vi "Periodic Tasks.vi"(8 "error in":errorcluster) -> ()   [LabVIEW 2016]
doc: "This VI runs in parallel to other tasks. It can contain as many user-defined periodic loops as you need. These can carry out PID or other sorts of timed response."
uses:
  <vilib>/Analysis/baseanly.llb/Mean (DBL).vi
  <vilib>/Rock Robotics/WPI/Utilities/WPI_GetSetVariantRefNum.vi
  LabView Programs/TestBot/global.vi
  <vilib>/Analysis/NI_AALBase.lvlib
panel:
  out "buffer":string
  out "error out 2":errorcluster
  out "X":i32
  out "Y":i32
  out "Width":i32
  out "Height":i32
  out "Area":dbl(graph)
  in  "Combo Box":string(combo)
  in  "Write":bool
  out "concatenated string":string
  in  "Flush":bool
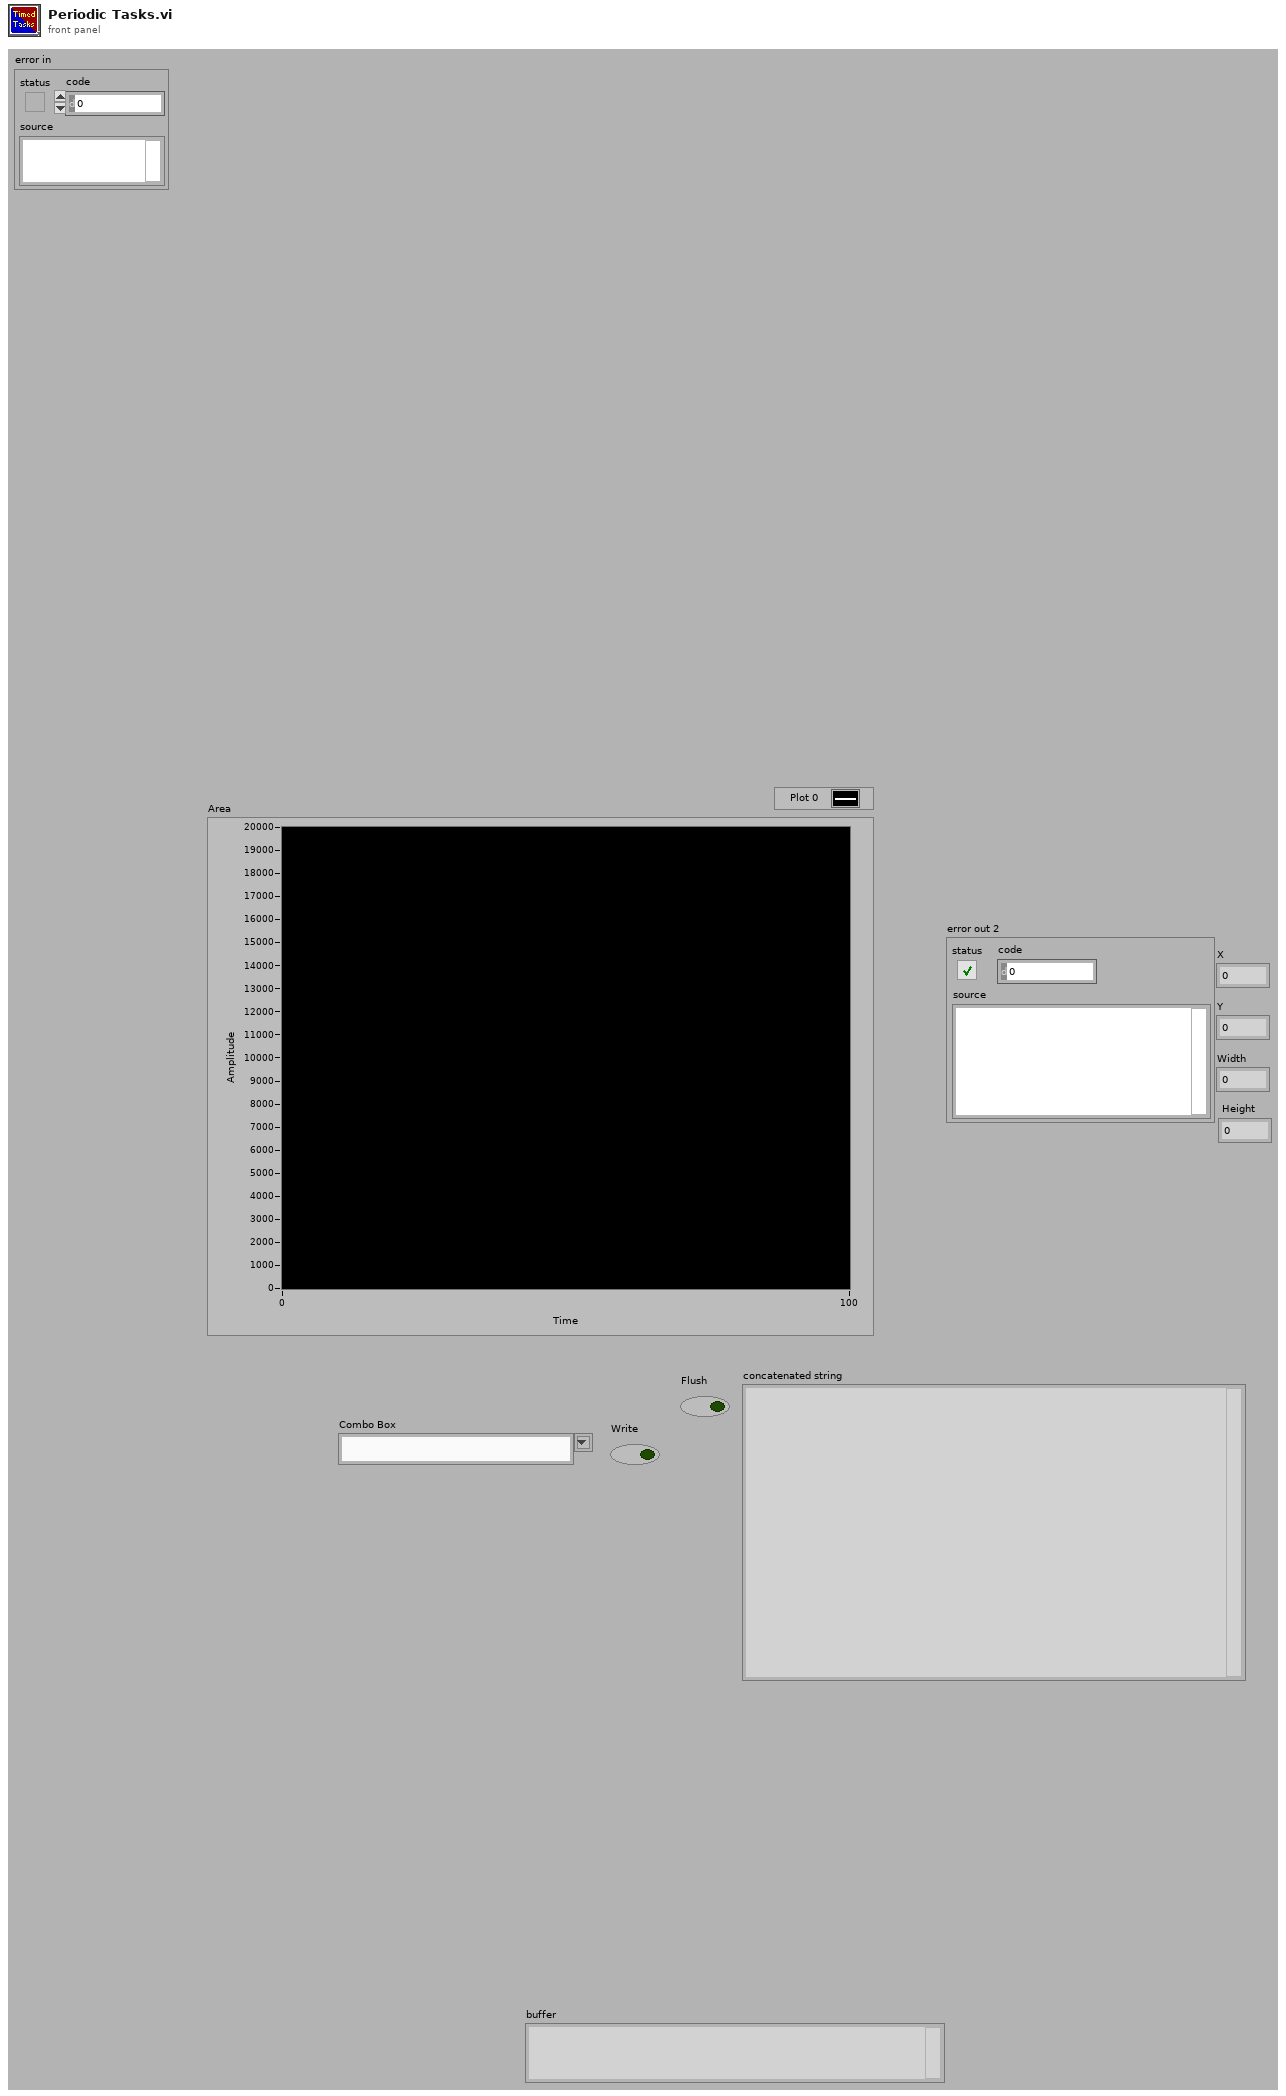
[diagram p1: front panel]
types:
  T1 = cluster{"buffer":string, "X":i32, "Y":i32, "Width":i32, "Height":i32, "Area":dbl}
  T2 = typedef "WPI_JoystickDevRef.ctl" = cluster{"Device":T3}
  T3 = typedef "WPI_JoystickDeviceEnum.ctl" = enum16{"USB 0", "USB 1", "USB 2", "USB 3", "USB 4", "USB 5"}
  T4 = typedef "WPI_SerialPortRef.ctl" = cluster{"DevStatus":errorcluster, "Serial Port Name":refnum<visa-resource-name>}
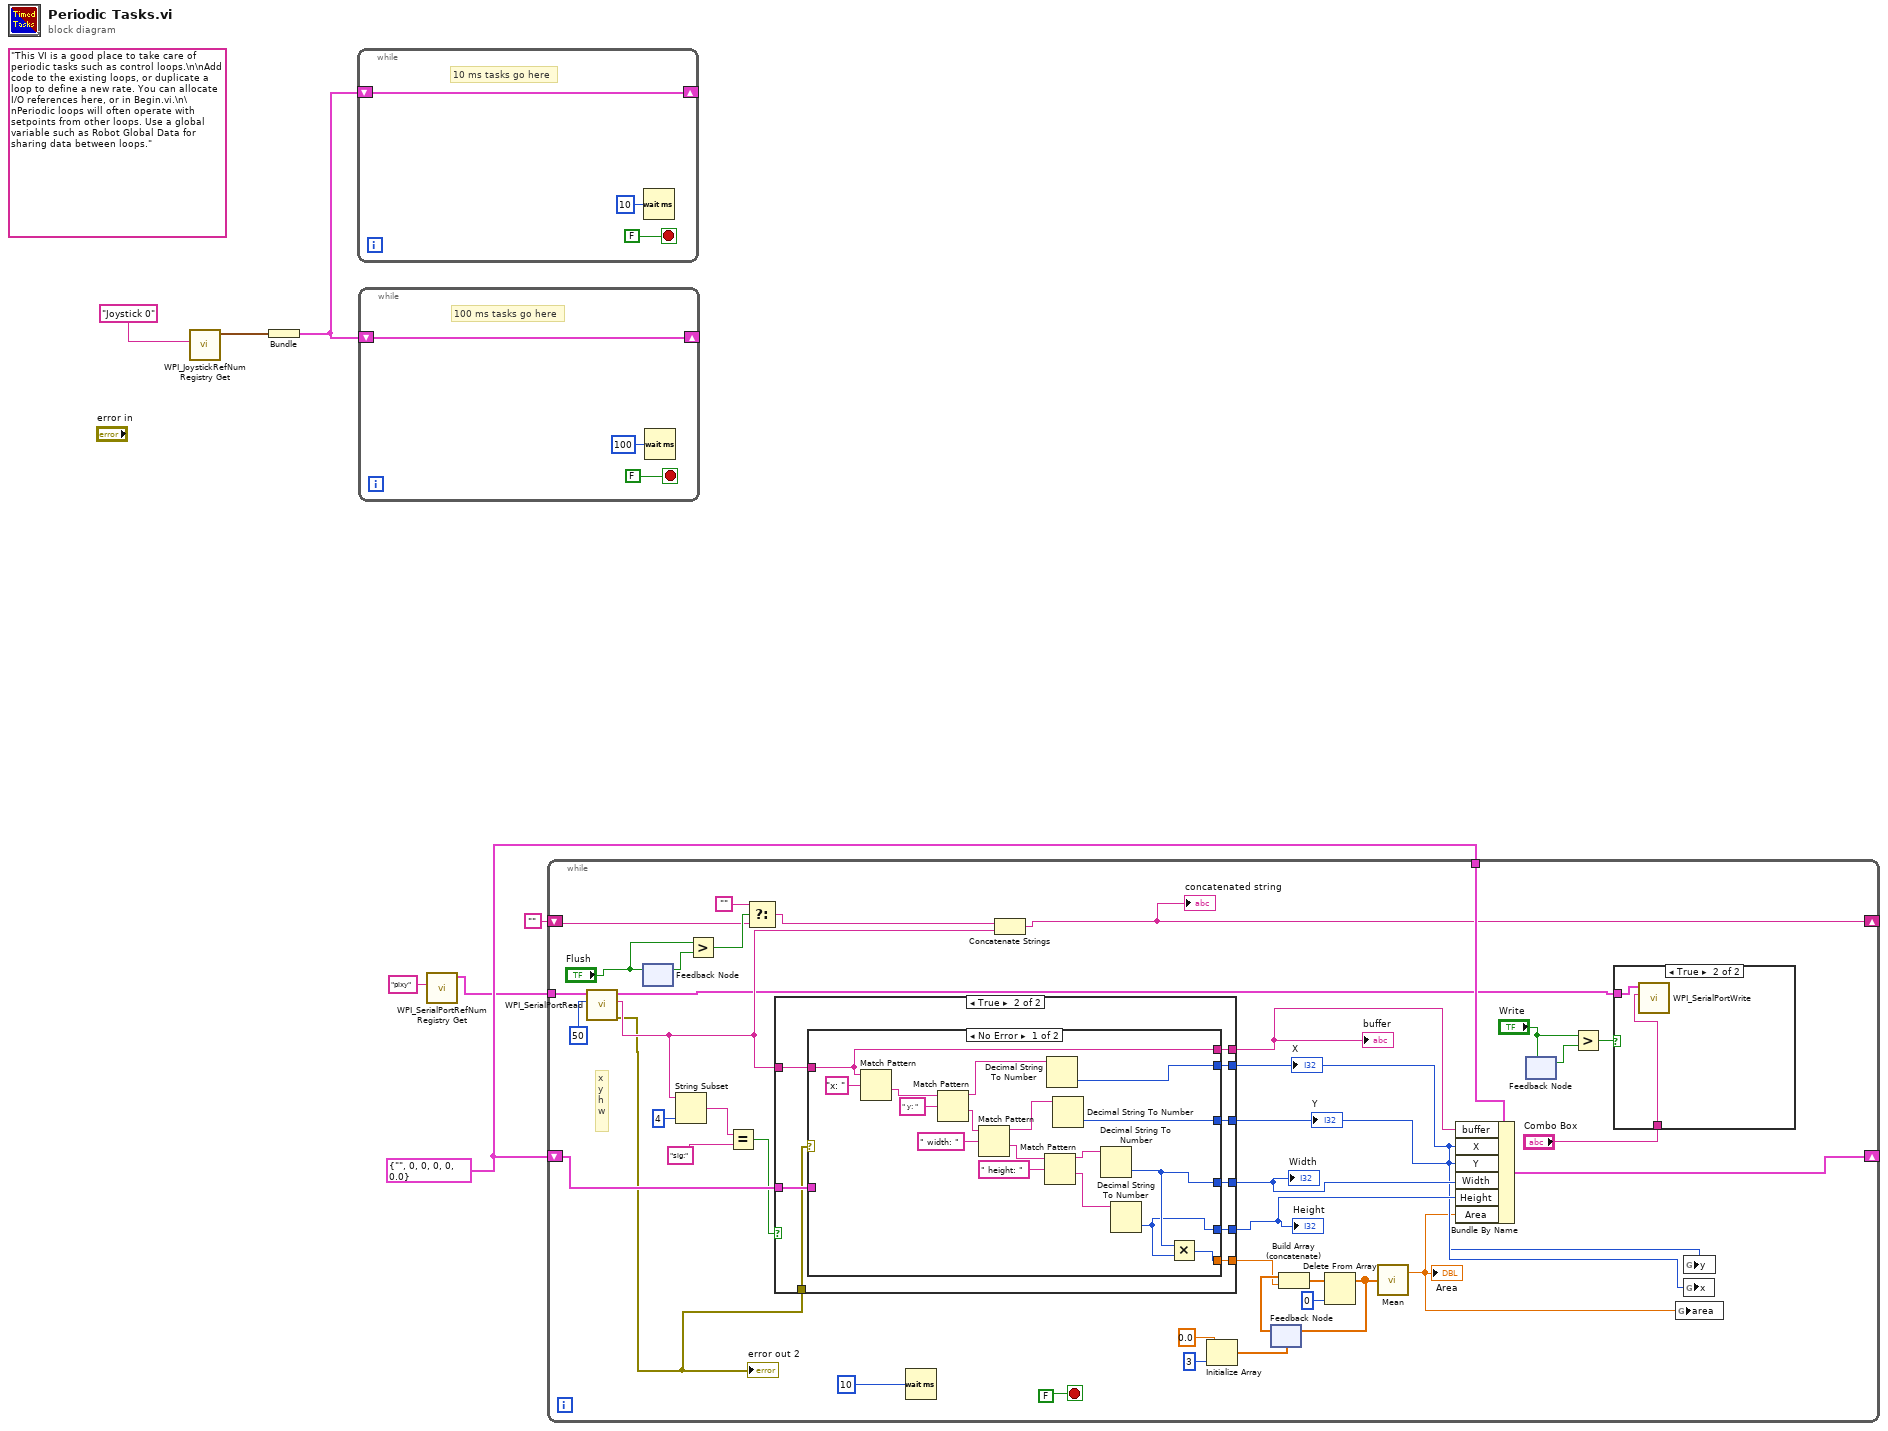
[diagram p0: block diagram]
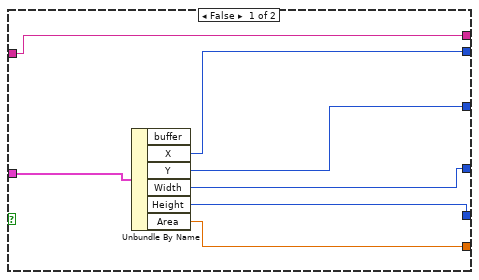
[diagram p2: hidden frame]
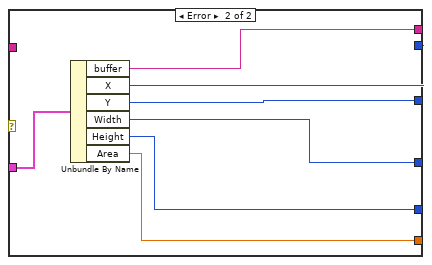
[diagram p3: hidden frame]
diagram:
  w4 = T1 {"buffer"="", "X"=0, "Y"=0, "Width"=0, "Height"=0, "Area"=0.0}
  (unwired) "This VI is a good place to take care of periodic tasks such as control loops.\n\nAdd code to the existing loops, or duplicate a loop to define a new rate. You can allocate I/O references here, or in Begin.vi.\n\nPeriodic loops will often operate with setpoints from other loops. Use a global variable such as Robot Global Data for sharing data between loops."
  n1 = call <vilib>:"WPI_JoystickRefNum Registry Get.vi"("refnum name"="Joystick 0") -> ("JoystickDevRef"=w6:T2)  [unwired: 1 in, 9 out]
  n2 = Bundle("JoystickDevRef"=w6) -> (w5:cluster{"JoystickDevRef":T2})  [unwired: 1 out]
  n3 = while {
    shift-right: [w8] -> _
    shift-left: w5 -> [w8]
    stop <- FALSE stop-if-true
    # "10 ms tasks go here"
    n4 = Wait (ms)(milliseconds to wait=u32 10) -> ()  [unwired: 1 out]
  }
  n5 = while {
    shift-right: [w11] -> _
    shift-left: w5 -> [w11]
    stop <- FALSE stop-if-true
    # "100 ms tasks go here"
    n6 = Wait (ms)(milliseconds to wait=u32 100) -> ()  [unwired: 1 out]
  }
  n7 = call <vilib>:"WPI_SerialPortRefNum Registry Get.vi"("refnum name"="pixy") -> ("SerialPortRef"=w2:T4)  [unwired: 9 in, 1 out]
  n8 = while {
    shift-right: [w50] -> _
    shift-left: w4 -> [w37]
    tunnel: w4 -> [w49]
    shift-right: [w28] -> _
    shift-left: "" -> [w24]
    tunnel: w2 -> [w17]
    stop <- FALSE ("stop") stop-if-true
    # "x\ny\nh\nw"
    n9 = call <vilib>:"WPI_SerialPortRead.vi"("Num Bytes to Read"=u32 50 ("byte count"), "SerialPortRef"=w17) -> ("error out"=w19:errorcluster, "Buffer"=w20:string, "SerialPortRef"=w18:T4)  [unwired: 7 in]
    "error out 2" <- w19
    n10 = feedback #1() -> (w27:bool)  [unwired: 1 in]
    n11 = feedback-in #1("Flush") -> ()
    n12 = String Subset(string=w20, length (rest)=4 ("length (rest)")) -> (substring=w33:string)  [unwired: 1 in]
    n13 = Greater?(x="Flush", y=w27) -> (0:w25:bool)
    n14 = Equal?(x=w33, y="sig:") -> (x = y?=w35:bool)
    n15 = Select(t="", s=w25, f=w24) -> (s? t:f=w22:string)
    n16 = case shown="True" w35 {
      tunnel: [w53 w68] -> w41
      tunnel: [w58 w67] -> w16
      tunnel: [w57 w66] -> w15
      tunnel: [w56 w65] -> w40
      tunnel: [w55 w64] -> w39
      tunnel: [w54 w63] -> w38
      tunnel: w20 -> [w53 w62]
      tunnel: w37 -> [w59 w61]
      tunnel: w19 -> [_ w60]
      frame False {
        n17 = Unbundle By Name(w59) -> ("X"=w58:i32, "Y"=w57:i32, "Width"=w56:i32, "Height"=w55:i32, "Area"=w54:dbl)  [unwired: 1 out]
      }
      frame True {
        n18 = case shown="No Error" w60 {
          tunnel: [w81 w87] -> w67
          tunnel: [w77 w88] -> w66
          tunnel: [w72 w89] -> w65
          tunnel: [w71 w90] -> w64
          tunnel: [w70 w91] -> w63
          tunnel: w61 -> [_ w92]
          tunnel: w62 -> [w69 _]
          tunnel: [w69 w86] -> w68
          frame No Error {
            n19 = Match Pattern(string=w69, regular expression="x: ") -> (after substring=w84:string)  [unwired: 1 in, 3 out]
            n20 = Match Pattern(string=w84, regular expression=" y: ") -> (before substring=w82:string, after substring=w80:string)  [unwired: 1 in, 2 out]
            n21 = Match Pattern(string=w80, regular expression=" width: ") -> (before substring=w78:string, after substring=w76:string)  [unwired: 1 in, 2 out]
            n22 = Match Pattern(string=w76, regular expression=" height: ") -> (before substring=w74:string, after substring=w73:string)  [unwired: 1 in, 2 out]
            n23 = Decimal String To Number(string=w82) -> (number=w81:i32)  [unwired: 2 in, 1 out]
            n24 = Decimal String To Number(string=w78) -> (number=w77:i32)  [unwired: 2 in, 1 out]
            n25 = Decimal String To Number(string=w74) -> (number=w72:i32)  [unwired: 2 in, 1 out]
            n26 = Decimal String To Number(string=w73) -> (number=w71:i32)  [unwired: 2 in, 1 out]
            n27 = Multiply(x=w72, y=w71) -> (x*y=w70:i32)
          }
          frame Error {
            n28 = Unbundle By Name(w92) -> ("buffer"=w86:string, "X"=w87:i32, "Y"=w88:i32, "Width"=w89:i32, "Height"=w90:i32, "Area"=w91:dbl)
          }
        }
      }
    }
    "buffer" <- w41
    "X" <- w16
    "Y" <- w15
    "Width" <- w40
    "Height" <- w39
    n29 = Wait (ms)(milliseconds to wait=u32 10) -> ()  [unwired: 1 out]
    n30 = Concatenate Strings(w22, w20) -> (w28:string)
    "concatenated string" <- w28
    n31 = Initialize Array(0.0 ("element"), 3 ("dimension size")) -> (w46:dbl[])
    n32 = feedback #2(w46) -> (w42:dbl[])
    n33 = Build Array (concatenate)(w42, w38) -> (w45:dbl[])
    n34 = Delete From Array(array=w45, index=0) -> (array with subset deleted=w44:dbl[])  [unwired: 1 in, 1 out]
    n35 = feedback-in #2(w44) -> ()
    n36 = call-poly <vilib>:"Mean.vi"("X"=w44) -> ("mean"=w14:dbl)  [unwired: 1 out]
    "Area" <- w14
    n37 = Bundle By Name(cluster=w49, "buffer"=w41, "X"=w16, "Y"=w15, "Width"=w40, "Height"=w39, "Area"=w14) -> (w50:T1)
    n38 = feedback-in #3("Write") -> ()
    n39 = feedback #3() -> (w30:bool)  [unwired: 1 in]
    n40 = Greater?(x="Write", y=w30) -> (0:w31:bool)
    n41 = case shown="True" w31 {
      tunnel: "Combo Box" -> [_ w93]
      tunnel: w18 -> [_ w94]
      frame False {
      }
      frame True {
        n42 = call <vilib>:"WPI_SerialPortWrite.vi"("Buffer"=w93, "SerialPortRef"=w94) -> ()  [unwired: 7 in, 3 out]
      }
    }
    n43 = global write "global.vi" "area"(w14) -> ()
    n44 = global write "global.vi" "y"(w15) -> ()
    n45 = global write "global.vi" "x"(w16) -> ()
  }
